vi "FPGA_96ch_Init.vi"() -> (0 "error out":errorcluster, 2 "FPGA VI Reference OUt":T1)   [LabVIEW 2011]
uses:
  FPGA_reference.ctl
  <vilib>/FPGAPlugInAG/PXI-7813R/niLvFpga_Open_PXI-7813R.vi
  <vilib>/Utility/error.llb/Error Cluster From Error Code.vi
  <vilib>/FPGAPlugInAG/PXI-7813R/niLvFpga_Reset_PXI-7813R.vi
  <vilib>/FPGAPlugInAG/PXI-7813R/niLvFpga_Run_PXI-7813R.vi
  <vilib>/rvi/interface/nirviOpenFPGA/nirviOpenFPGA.xnode
  FPGA Bitfiles/FPGA96chmodular3_FPGATarget_fpga96ch-Maindea_7F81622F.lvbitx
  fpga_96ch-Main_dead_pixels.vi
  <vilib>/rvi/interface/nirviMethod/nirviMethod.xnode
  <vilib>/FPGAPlugInAG/PXI-7813R/niLvFpga_ConfigureFifo_PXI-7813R.vi
  <vilib>/rvi/errors/niLvFpgaMergeErrorWithErrorCode.vi
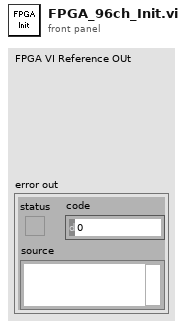
[diagram p1: front panel]
types:
  T1 = typedef "FPGA_reference.ctl" = refnum<k20>
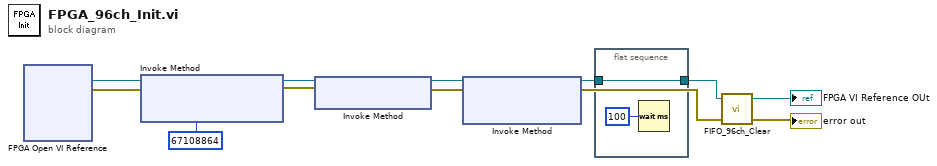
[diagram p0: block diagram]
diagram:
  n1 = xnode "FPGA Open VI Reference"() -> ("FPGA VI Reference Out"=w4:refnum<k20>, "error out"=w5:errorcluster)  [unwired: 2 in]
  n2 = xnode "Invoke Method"("FPGA VI Reference In"=w4, "error in"=w5, "Depth"=u32 67108864) -> ("FPGA VI Reference Out"=w8:refnum<k20>, "error out"=w7:errorcluster)
  n3 = xnode "Invoke Method"("FPGA VI Reference In"=w8, "error in"=w7) -> ("FPGA VI Reference Out"=w10:refnum<k20>, "error out"=w9:errorcluster)
  n4 = xnode "Invoke Method"("FPGA VI Reference In"=w10, "error in"=w9) -> ("FPGA VI Reference Out"=w3:refnum<k20>, "error out"=w12:errorcluster)  [unwired: 1 in]
  n5 = flat-sequence {
    tunnel: w3 -> [w13]
    tunnel: [w13] -> w2
    frame #0 {
      n6 = Wait (ms)(milliseconds to wait=u32 100) -> ()  [unwired: 1 out]
    }
  }
  n7 = call "FIFO_96ch_Clear.vi"("error in"=w12, "FPGA VI Reference In"=w2) -> ("error out"=→"error out":errorcluster, "FPGA VI Reference Out"=→"FPGA VI Reference OUt":T1)  [unwired: 2 in]
